vi "ForExample.vi"() -> ()   [LabVIEW 2018]
uses:
  <vilib>/Analysis/1siggen.llb/Ramp Pattern by Samples.vi
  <vilib>/Analysis/NI_AALBase.lvlib
panel:
  out "Ramp Pattern":dbl[](array[numeric])
  out "Array":string[](array[string])
  in  "Numeric":dbl
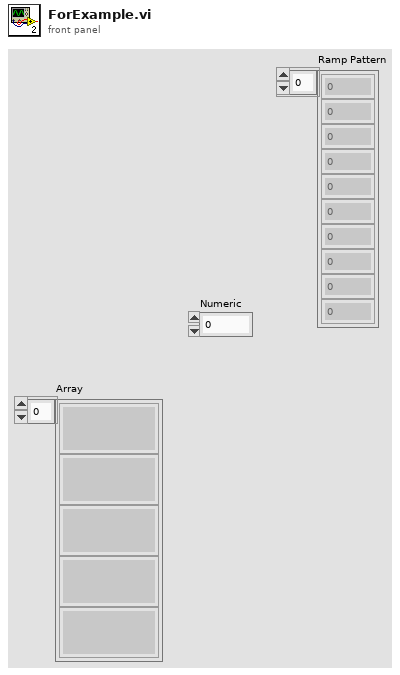
[diagram p1: front panel]
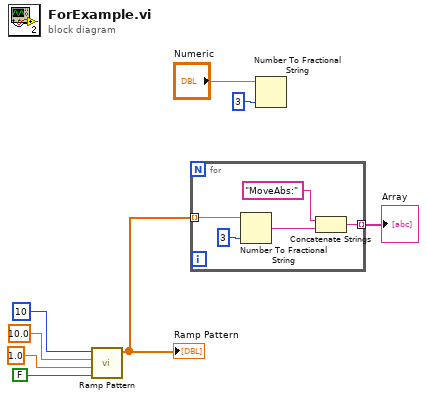
[diagram p0: block diagram]
diagram:
  n1 = call-poly <vilib>:"Ramp Pattern.vi"("exclude end?"=FALSE, "start"=1.0, "end"=10.0 ("start"), "samples"=10) -> ("Ramp Pattern"=w1:dbl[])  [unwired: 6 in, 1 out]
  "Ramp Pattern" <- w1
  n2 = for {
    tunnel: [w10] -> w6 mode=indexing
    tunnel: w1 -> [w9] mode=indexing
    n3 = Number To Fractional String(number=w9, precision (6)=i16 3) -> (F-format string=w11:string)  [unwired: 2 in]
    n4 = Concatenate Strings("MoveAbs:", w11) -> (w10:string)
  }
  "Array" <- w6
  n5 = Number To Fractional String(number="Numeric", precision (6)=i16 3) -> ()  [unwired: 2 in, 1 out]
